vi "Host Application (Main).vi"() -> ()   [LabVIEW 2015]
doc: "Shared Variable Benchmarking Utility - Allows for the programmatic benchmarking of shared variable perfomance from single host to single target."
uses:
  Type Defs/Sequence Parameters.ctl
  Type Defs/Target Type.ctl
  Type Defs/Variable Data Type.ctl
  Type Defs/Target Config Cluster.ctl
  Type Defs/RT Target Type.ctl
  Type Defs/Control Refs.ctl
  SV B-M (Host) Class/SV B-M (Host).lvclass
panel:
  in  "Tab Control":T1(tab)=enum."Benchmark Utility"
  in  "Abort Config":bool
  in  "Run Config":bool
  out "Config Console":string="Waiting..."
  in  "Targets to Configure":T2[](array[typedef])
  out "Test #":string
  in  "Load":bool
  in  "Save":bool
  in  "Delete":bool
  in  "Copy":bool
  in  "Insert After":bool
  in  "Insert Before":bool
  in  "Seq Parameters":T4[](array[typedef]) {"# of Variables per Library" items=["50"=50, "100"=100, "150"=150, "200"=200, "250"=250, "300"=300, "350"=350, "400"=400, "450"=450, "500"=500]; "Delta" min=50 max=1000000 step=50; "Ceiling" min=50 max=1000000 step=50; "Floor" min=50 max=1000000 step=50}
  in  "Abort BM":bool
  in  "Run BM":bool
  out "Test in Progress :":string
  in  "MC Listbox":i32(listbox)=-1
  in  "Load":bool
  in  "Sequence Directory":path
  out "Config Params":T4[](array[typedef]) {"# of Variables per Library" items=["50"=50, "100"=100, "150"=150, "200"=200, "250"=250, "300"=300, "350"=350, "400"=400, "450"=450, "500"=500]; "Delta" min=50 max=1000000 step=50; "Ceiling" min=50 max=1000000 step=50; "Floor" min=50 max=1000000 step=50}
  out "CPU Load Data":cluster{dbl[], dbl[]}(graph)
  # "Shared Variable Benchmarking Utility"
  # "Target IP Address"
  # "Target Type"
  # "Username"
  # "Password"
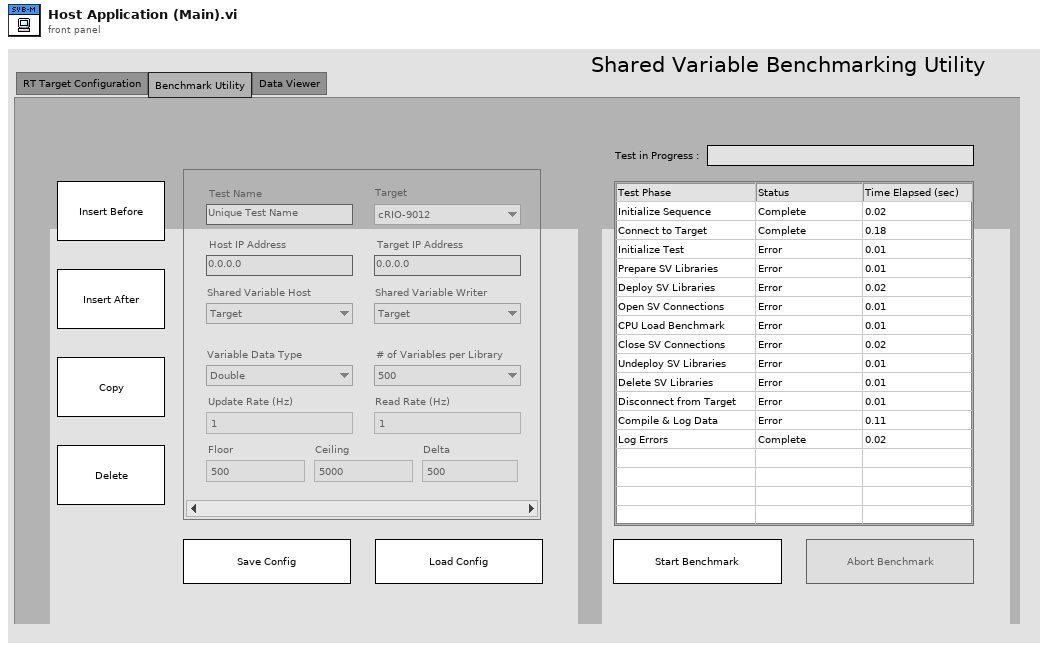
[diagram p1: front panel]
types:
  T1 = enum32{"RT Target Configuration", "Benchmark Utility", "Data Viewer"}
  T2 = typedef "Target Config Cluster.ctl" = cluster{"IP Address":string, "Target":T3, "Username":string, "Password":string}
  T3 = typedef "RT Target Type.ctl" = enum16{"cRIO-9012", "cRIO-9014", "cRIO-9022", "cRIO-9023", "cRIO-9024", "cRIO-9025", "cRIO-9068", "cRIO-9073", "cRIO-9074", "cRIO-9075", "cRIO-9076", "cRIO-9081", "cRIO-9082", "myRIO-1900", "myRIO-1950", "PXI-8101", "PXI-8115", "PXI-8119", "PXI-8820", "PXIe-8100", "PXIe-8101", "PXIe-8133", "PXIe-8135", "PXIe-8820", "sbRIO-9605", "sbRIO-9606", "sbRIO-9623", "sbRIO-9626", "sbRIO-9633", "sbRIO-9636", "Unlisted (Linux-RT)", "Unlisted (PharLap)", "Unlisted (VxWorks)"}
  T4 = typedef "Sequence Parameters.ctl" = cluster{"Test Name":string, "Target":T5, "Host IP Address":string, "Target IP Address":string, "Shared Variable Host":enum16{"Target", "Host"}, "Shared Variable Writer":enum16{"Target", "Host"}, "Variable Data Type":T6, "# of Variables per Library":u16, "Update Rate (Hz)":dbl, "Read Rate (Hz)":dbl, "Floor":u32, "Ceiling":u32, "Delta":u32}
  T5 = typedef "Target Type.ctl" = enum16{"cRIO-9012", "cRIO-9014", "cRIO-9022", "cRIO-9023", "cRIO-9024", "cRIO-9025", "cRIO-9068", "cRIO-9073", "cRIO-9074", "cRIO-9075", "cRIO-9076", "cRIO-9081", "cRIO-9082", "myRIO-1900", "myRIO-1950", "PXI-8101", "PXI-8115", "PXI-8119", "PXI-8820", "PXIe-8100", "PXIe-8101", "PXIe-8133", "PXIe-8135", "PXIe-8820", "sbRIO-9605", "sbRIO-9606", "sbRIO-9623", "sbRIO-9626", "sbRIO-9633", "sbRIO-9636", "Unlisted (Linux-RT)", "Unlisted (PharLap)", "Unlisted (VxWorks)", "Windows Target"}
  T6 = typedef "Variable Data Type.ctl" = enum16{"U8", "U16", "U32", "U64", "I8", "I16", "I32", "I64", "Single", "Double", "Boolean", "String"}
  T7 = enum16{"BM Init", "BM Run", "BM End", "Config Init", "Config Run", "Config End"}
  T8 = typedef "Control Refs.ctl" = cluster{"Save":refnum<vi>, "Load":refnum<vi>, "Delete":refnum<vi>, "Copy":refnum<vi>, "Insert Before":refnum<vi>, "Insert After":refnum<vi>, "Run BM":refnum<vi>, "Abort BM":refnum<vi>, "Run Config":refnum<vi>, "Abort Config":refnum<vi>, "Seq Parameters":refnum<vi>, "Target Config":refnum<vi>}
  T9 = typedef "Sequence Parameters Ref.ctl" = refnum<vi>
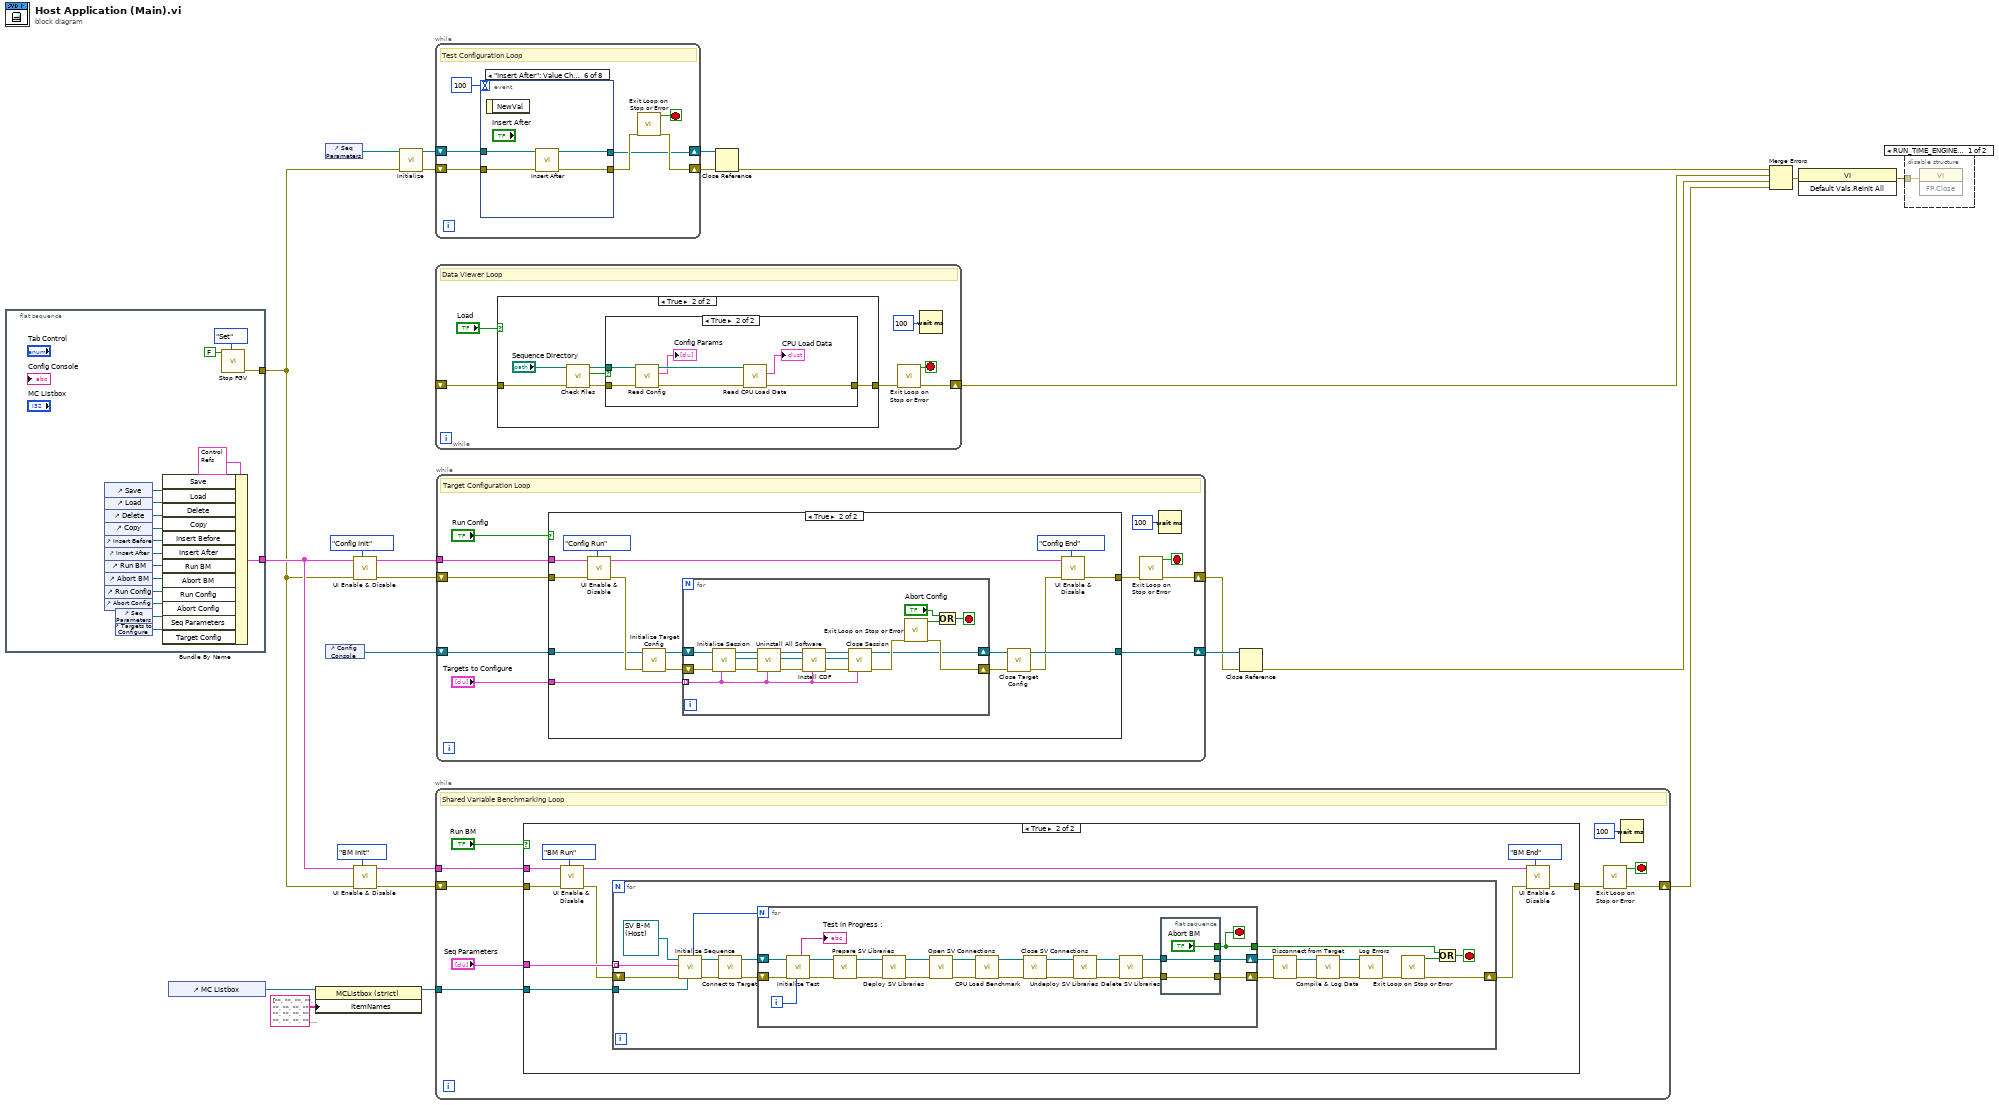
[diagram p0: block diagram]
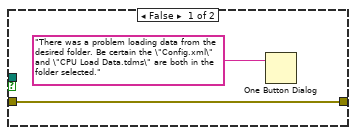
[diagram p3: hidden frame]
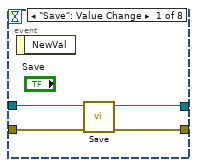
[diagram p7: hidden frame]
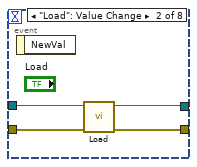
[diagram p8: hidden frame]
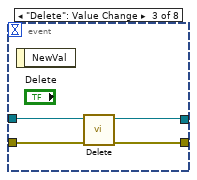
[diagram p9: hidden frame]
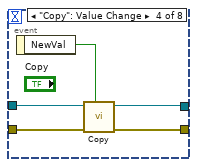
[diagram p10: hidden frame]
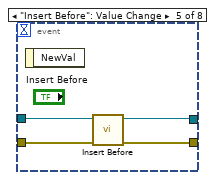
[diagram p11: hidden frame]
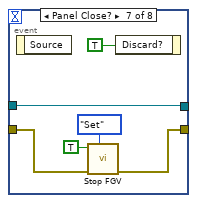
[diagram p12: hidden frame]
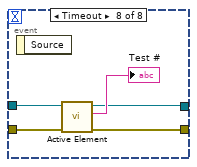
[diagram p13: hidden frame]
diagram:
  n1 = flat-sequence {
    tunnel: [w27] -> w4
    tunnel: [w26] -> w14
    frame #0 {
      n2 = control-ref of="Save"() -> (w40:refnum<vi>)
      n3 = control-ref of="Load"() -> (w39:refnum<vi>)
      n4 = control-ref of="Delete"() -> (w38:refnum<vi>)
      n5 = control-ref of="Copy"() -> (w37:refnum<vi>)
      n6 = control-ref of="Insert Before"() -> (w36:refnum<vi>)
      n7 = control-ref of="Insert After"() -> (w35:refnum<vi>)
      n8 = control-ref of="Run BM"() -> (w34:refnum<vi>)
      n9 = control-ref of="Abort BM"() -> (w33:refnum<vi>)
      n10 = control-ref of="Run Config"() -> (w32:refnum<vi>)
      n11 = control-ref of="Abort Config"() -> (w31:refnum<vi>)
      n12 = control-ref of="Seq Parameters"() -> (w30:refnum<vi>)
      n13 = control-ref of="Targets to Configure"() -> (w28:refnum<vi>)
      n14 = Bundle By Name(cluster=T8 {"Save"=refnum, "Load"=refnum, "Delete"=refnum, "Copy"=refnum, "Insert Before"=refnum, "Insert After"=refnum, "Run BM"=refnum, "Abort BM"=refnum, "Run Config"=refnum, "Abort Config"=refnum, "Seq Parameters"=refnum, "Target Config"=refnum} ("Cluster"), "Save"=w40, "Load"=w39, "Delete"=w38, "Copy"=w37, "Insert Before"=w36, "Insert After"=w35, "Run BM"=w34, "Abort BM"=w33, "Run Config"=w32, "Abort Config"=w31, "Seq Parameters"=w30, "Target Config"=w28) -> (w26:T8)
      n15 = call "Stop FGV.vi"("Mode"=enum16{"Set", "Get"}."Set", "Set Stop Condition"=FALSE) -> ("error out (no error)"=w27:errorcluster)  [unwired: 8 in, 1 out]
    }
  }
  n16 = control-ref of="MC Listbox"() -> (w8:refnum<vi>)
  n17 = property class="MCListbox (strict)"(reference=w8, "ItemNames"=string[][] [["", "", "", "", "", "", "", "", "", "", "", "", "", "", "", "", "", "", "", "", ""], ["", "", "", "", "", "", "", "", "", "", "", "", "", "", "", "", "", "", "", "", ""], ["", "", "", "", "", "", "", "", "", "", "", "", "", "", "", "", "", "", "", "", ""], ["", "", "", "", "", "", "", "", "", "", "", "", "", "", "", "", "", "", "", "", ""], ["", "", "", "", "", "", "", "", "", "", "", "", "", "", "", "", "", "", "", "", ""], ["", "", "", "", "", "", "", "", "", "", "", "", "", "", "", "", "", "", "", "", ""], ["", "", "", "", "", "", "", "", "", "", "", "", "", "", "", "", "", "", "", "", ""], ["", "", "", "", "", "", "", "", "", "", "", "", "", "", "", "", "", "", "", "", ""], ["", "", "", "", "", "", "", "", "", "", "", "", "", "", "", "", "", "", "", "", ""], ["", "", "", "", "", "", "", "", "", "", "", "", "", "", "", "", "", "", "", "", ""], ["", "", "", "", "", "", "", "", "", "", "", "", "", "", "", "", "", "", "", "", ""], ["", "", "", "", "", "", "", "", "", "", "", "", "", "", "", "", "", "", "", "", ""], ["", "", "", "", "", "", "", "", "", "", "", "", "", "", "", "", "", "", "", "", ""], ["", "", "", "", "", "", "", "", "", "", "", "", "", "", "", "", "", "", "", "", ""], ["", "", "", "", "", "", "", "", "", "", "", "", "", "", "", "", "", "", "", "", ""], ["", "", "", "", "", "", "", "", "", "", "", "", "", "", "", "", "", "", "", "", ""], ["", "", "", "", "", "", "", "", "", "", "", "", "", "", "", "", "", "", "", "", ""], ["", "", "", "", "", "", "", "", "", "", "", "", "", "", "", "", "", "", "", "", ""], ["", "", "", "", "", "", "", "", "", "", "", "", "", "", "", "", "", "", "", "", ""], ["", "", "", "", "", "", "", "", "", "", "", "", "", "", "", "", "", "", "", "", ""], ["", "", "", "", "", "", "", "", "", "", "", "", "", "", "", "", "", "", "", "", "."]] ("Item Names")) -> (reference out=w6:refnum<vi>)  [unwired: 1 in, 1 out]
  n18 = control-ref of="Config Console"() -> (w13:refnum<vi>)
  n19 = control-ref of="Seq Parameters"() -> (w5:refnum<vi>)
  n20 = call "UI Enable & Disable.vi"("Mode"=T7."Config Init", "error in (no error)"=w4, "Ctl Refs In"=w14) -> ("error out"=w15:errorcluster, "Ctl Refs Out"=w16:T8)  [unwired: 7 in]
  n21 = call "UI Enable & Disable.vi"("Mode"=T7."BM Init", "error in (no error)"=w4, "Ctl Refs In"=w14) -> ("error out"=w20:errorcluster, "Ctl Refs Out"=w18:T8)  [unwired: 7 in]
  n22 = call "Initialize.vi"("error in (no error)"=w4, "Test Configs In"=w5) -> ("error out"=w25:errorcluster, "Test Configs Out"=w22:T9)  [unwired: 8 in]
  n23 = while {
    shift-right: [w46] -> w24
    shift-left: w25 -> [w49]
    shift-right: [w43] -> w21
    shift-left: w22 -> [w44]
    stop <- w45 stop-if-true
    # "Test Configuration Loop"
    n24 = event shown="[5] \"Insert After\": Value Change" {
      selector: _ -> [_ _ _ _ _ _ _ _]
      dyn-events: _ -> [_ _ _ _ _ _ _ _]
      timeout: 100 -> [_ _ _ _ _ _ _ _]
      tunnel: w49 -> [w53 w57 w61 w66 w70 w74 w79 w85]
      tunnel: [w52 w56 w60 w65 w69 w73 w78 w84] -> w47
      tunnel: w44 -> [w51 w55 w59 w63 w68 w72 w75 w82]
      tunnel: [w50 w54 w58 w62 w67 w71 w75 w81] -> w43
      event "Save": Value Change {
        n25 = event-data() -> ()  [unwired: 1 in, 1 out]
        n26 = call "Save.vi"("error in (no error)"=w53, "Test Configs In"=w51) -> ("error out"=w52:errorcluster, "Test Configs Out"=w50:T9)  [unwired: 8 in]
      }
      event "Load": Value Change {
        n27 = event-data() -> ()  [unwired: 1 in, 1 out]
        n28 = call "Load.vi"("error in (no error)"=w57, "Test Configs In"=w55) -> ("error out"=w56:errorcluster, "Test Configs Out"=w54:T9)  [unwired: 8 in]
      }
      event "Delete": Value Change {
        n29 = event-data() -> ()  [unwired: 1 in, 1 out]
        n30 = call "Delete.vi"("error in (no error)"=w61, "Test Configs In"=w59) -> ("error out"=w60:errorcluster, "Test Configs Out"=w58:T9)  [unwired: 8 in]
      }
      event "Copy": Value Change {
        n31 = event-data() -> ("NewVal"=w64:bool)  [unwired: 1 in]
        n32 = call "Copy.vi"("Copy Enabled?"=w64, "error in (no error)"=w66, "Test Configs In"=w63) -> ("error out"=w65:errorcluster, "Test Configs Out"=w62:T9)  [unwired: 7 in]
      }
      event "Insert Before": Value Change {
        n33 = event-data() -> ()  [unwired: 1 in, 1 out]
        n34 = call "Insert Before.vi"("error in (no error)"=w70, "Test Configs In"=w68) -> ("error out"=w69:errorcluster, "Test Configs Out"=w67:T9)  [unwired: 8 in]
      }
      event "Insert After": Value Change {
        n35 = event-data() -> ()  [unwired: 1 in, 1 out]
        n36 = call "Insert After.vi"("error in (no error)"=w74, "Test Configs In"=w72) -> ("error out"=w73:errorcluster, "Test Configs Out"=w71:T9)  [unwired: 8 in]
      }
      event Panel Close? {
        n37 = event-data() -> ()  [unwired: 1 in, 1 out]
        n38 = call "Stop FGV.vi"("Mode"=enum16{"Set", "Get"}."Set", "error in (no error)"=w79, "Set Stop Condition"=TRUE) -> ("error out (no error)"=w78:errorcluster)  [unwired: 7 in, 1 out]
        n39 = event-data("Discard?"=TRUE) -> ()  [unwired: 1 in, 1 out]
      }
      event Timeout {
        n40 = event-data() -> ()  [unwired: 1 in, 1 out]
        n41 = call "Active Element.vi"("error in (no error)"=w85, "Test Configs In"=w82) -> ("error out"=w84:errorcluster, "Active Test"=→"Test #":string, "Test Configs Out"=w81:T9)  [unwired: 7 in]
      }
    }
    n42 = call "Exit Loop on Stop or Error.vi"("error in (no error)"=w47) -> ("error out"=w46:errorcluster, "Exit?"=w45:bool)  [unwired: 9 in]
  }
  n43 = while {
    shift-right: [w87] -> w1
    shift-left: _ -> [w90]
    stop <- w88 stop-if-true
    # "Data Viewer Loop"
    n44 = case shown="True" "Load" {
      tunnel: w90 -> [w92 w97]
      tunnel: [w92 w98] -> w89
      frame False {
      }
      frame True {
        n45 = call "Check Files.vi"("error in (no error)"=w97, "Sequence Directory In"="Sequence Directory") -> ("error out"=w95:errorcluster, "Files Valid?"=w94:bool, "Sequence Directory Out"=w93:path)  [unwired: 7 in]
        n46 = case shown="True" w94 {
          tunnel: [w100 w106] -> w98
          tunnel: w95 -> [w100 w105]
          tunnel: w93 -> [_ w104]
          frame False {
            n47 = One Button Dialog(message="There was a problem loading data from the desired folder. Be certain the \"Config.xml\" and \"CPU Load Data.tdms\" are both in the folder selected.") -> ()  [unwired: 1 in, 1 out]
          }
          frame True {
            n48 = call "Read Config.vi"("error in (no error)"=w105, "Sequence Directory"=w104) -> ("error out"=w107:errorcluster, "Sequence Parameters"=→"Config Params":T4[], "Sequence Directory Out"=w103:path)  [unwired: 7 in]
            n49 = call "Read CPU Load Data.vi"("error in (no error)"=w107, "Sequence Directory In"=w103) -> ("error out"=w106:errorcluster, "XY Graph Data"=→"CPU Load Data":cluster{dbl[], dbl[]})  [unwired: 7 in, 1 out]
          }
        }
      }
    }
    n50 = call "Exit Loop on Stop or Error.vi"("error in (no error)"=w89) -> ("error out"=w87:errorcluster, "Exit?"=w88:bool)  [unwired: 9 in]
    n51 = Wait (ms)(milliseconds to wait=u32 100) -> ()  [unwired: 1 out]
  }
  n52 = while {
    shift-right: [w108] -> w10
    shift-left: w20 -> [w115]
    tunnel: w18 -> [w112]
    tunnel: w6 -> [w110]
    stop <- w113 stop-if-true
    # "Shared Variable Benchmarking Loop"
    n53 = case shown="True" "Run BM" {
      tunnel: w115 -> [w117 w127]
      tunnel: w112 -> [_ w126]
      tunnel: "Seq Parameters" -> [_ w122]
      tunnel: w110 -> [_ w120]
      tunnel: [w117 w118] -> w109
      frame False {
      }
      frame True {
        n54 = call "UI Enable & Disable.vi"("Mode"=T7."BM Run", "error in (no error)"=w127, "Ctl Refs In"=w126) -> ("error out"=w121:errorcluster, "Ctl Refs Out"=w124:T8)  [unwired: 7 in]
        n55 = for {
          tunnel: w122 -> [w147] mode=indexing
          shift-right: [w143] -> w119
          shift-left: w121 -> [w146]
          tunnel: w120 -> [w144]
          stop <- w141 stop-if-true
          n56 = call "Initialize Sequence.vi"("Listbox Ref In"=w144, "error in (no error)"=w146, "Seq Parameters"=w147, "SV B-M in"=refnum<class "SV B-M (Host).lvclass"> refnum ("SV B-M.lvclass")) -> ("error out"=w137:errorcluster, "SV B-M out"=w139:refnum<class "SV B-M (Host).lvclass">, "# of Tests"=w140:i32)  [unwired: 5 in]
          n57 = call "Connect to Target.vi"("error in (no error)"=w137, "SV B-M (Host) in"=w139) -> ("error out"=w136:errorcluster, "SV B-M (Host) out"=w138:refnum<class "SV B-M (Host).lvclass">)  [unwired: 8 in]
          n58 = for {
            N: w140 -> [_]
            shift-right: [w149] -> w133
            shift-left: w136 -> [w170]
            shift-right: [w151] -> w134
            shift-left: w138 -> [w169]
            tunnel: [w148] -> w132
            i -> [w167]
            stop <- w148 stop-if-true
            n59 = call "Initialize Test.vi"("Test Index"=w167, "error in (no error)"=w170, "SV B-M in"=w169) -> ("error out"=w165:errorcluster, "SV B-M out"=w166:refnum<class "SV B-M (Host).lvclass">, "Test In Progress"=→"Test in Progress :":string)  [unwired: 6 in]
            n60 = call "Prepare SV Libraries.vi"("error in (no error)"=w165, "SV B-M in"=w166) -> ("error out"=w163:errorcluster, "SV B-M out"=w164:refnum<class "SV B-M (Host).lvclass">)  [unwired: 8 in]
            n61 = call "Deploy SV Libraries.vi"("error in (no error)"=w163, "SV B-M in"=w164) -> ("error out"=w159:errorcluster, "SV B-M out"=w160:refnum<class "SV B-M (Host).lvclass">)  [unwired: 8 in]
            n62 = call "Open SV Connections.vi"("error in (no error)"=w159, "SV B-M (Host) in"=w160) -> ("error out"=w155:errorcluster, "SV B-M (Host) out"=w156:refnum<class "SV B-M (Host).lvclass">)  [unwired: 8 in]
            n63 = call "CPU Load Benchmark.vi"("error in (no error)"=w155, "SV B-M (Host) in"=w156) -> ("error out"=w153:errorcluster, "SV B-M (Host) out"=w154:refnum<class "SV B-M (Host).lvclass">)  [unwired: 8 in]
            n64 = call "Close SV Connections.vi"("error in (no error)"=w153, "SV B-M (Host) in"=w154) -> ("error out"=w157:errorcluster, "SV B-M (Host) out"=w158:refnum<class "SV B-M (Host).lvclass">)  [unwired: 8 in]
            n65 = call "Undeploy SV Libraries.vi"("error in (no error)"=w157, "SV B-M in"=w158) -> ("error out"=w161:errorcluster, "SV B-M out"=w162:refnum<class "SV B-M (Host).lvclass">)  [unwired: 8 in]
            n66 = call "Delete SV Libraries.vi"("error in (no error)"=w161, "SV B-M (Host) in"=w162) -> ("error out"=w150:errorcluster, "SV B-M (Host) out"=w152:refnum<class "SV B-M (Host).lvclass">)  [unwired: 8 in]
            n67 = flat-sequence {
              tunnel: ["Abort BM"] -> w148
              tunnel: w152 -> [w172]
              tunnel: [w172] -> w151
              tunnel: [w171] -> w149
              tunnel: w150 -> [w171]
              frame #0 {
              }
            }
          }
          n68 = call "Disconnect from Target.vi"("error in (no error)"=w133, "SV B-M (Host) in"=w134) -> ("error out"=w131:errorcluster, "SV B-M (Host) out"=w130:refnum<class "SV B-M (Host).lvclass">)  [unwired: 8 in]
          n69 = call "Compile & Log Data.vi"("error in (no error)"=w131, "SV B-M (Host) in"=w130) -> ("error out"=w128:errorcluster, "SV B-M (Host) out"=w129:refnum<class "SV B-M (Host).lvclass">)  [unwired: 8 in]
          n70 = call "Log Errors.vi"("error in (no error)"=w128, "SV B-M (Host) in"=w129) -> ("error out"=w135:errorcluster)  [unwired: 9 in]
          n71 = call "Exit Loop on Stop or Error.vi"("error in (no error)"=w135) -> ("error out"=w143:errorcluster, "Exit?"=w142:bool)  [unwired: 9 in]
          n72 = Or(x=w132, y=w142) -> (x .or. y?=w141:bool)
        }
        n73 = call "UI Enable & Disable.vi"("Mode"=T7."BM End", "error in (no error)"=w119, "Ctl Refs In"=w124) -> ("error out"=w118:errorcluster)  [unwired: 7 in, 1 out]
      }
    }
    n74 = call "Exit Loop on Stop or Error.vi"("error in (no error)"=w109) -> ("error out"=w108:errorcluster, "Exit?"=w113:bool)  [unwired: 9 in]
    n75 = Wait (ms)(milliseconds to wait=u32 100) -> ()  [unwired: 1 out]
  }
  n76 = while {
    shift-right: [w178] -> w11
    shift-left: w15 -> [w183]
    tunnel: w16 -> [w180]
    shift-right: [w174] -> w12
    shift-left: w13 -> [w176]
    stop <- w181 stop-if-true
    # "Target Configuration Loop"
    n77 = case shown="True" "Run Config" {
      tunnel: w183 -> [w185 w200]
      tunnel: w180 -> [_ w199]
      tunnel: [w185 w195] -> w179
      tunnel: w176 -> [w184 w192]
      tunnel: "Targets to Configure" -> [_ w190]
      tunnel: [w184 w187] -> w174
      frame False {
      }
      frame True {
        n78 = call "UI Enable & Disable.vi"("Mode"=T7."Config Run", "error in (no error)"=w200, "Ctl Refs In"=w199) -> ("error out"=w194:errorcluster, "Ctl Refs Out"=w197:T8)  [unwired: 7 in]
        n79 = call "Initialize Target Config.vi"("error in (no error)"=w194, "Console Ref In"=w192) -> ("error out"=w193:errorcluster, "Console Ref Out"=w191:refnum<vi>)  [unwired: 8 in]
        n80 = for {
          shift-right: [w218] -> w188
          shift-left: w193 -> [w207]
          shift-right: [w201] -> w189
          shift-left: w191 -> [w208]
          tunnel: w190 -> [w203] mode=indexing
          stop <- w216 stop-if-true
          n81 = call "Initialize Session.vi"("Target Config"=w203, "error in (no error)"=w207, "Console Ref In"=w208) -> ("error out"=w206:errorcluster, "Sys Cfg Session Out"=w213:refnum<k21>, "Console Ref Out"=w214:refnum<vi>)  [unwired: 6 in]
          n82 = call "Uninstall All Software.vi"("Target Config"=w203, "error in (no error)"=w206, "Sys Cfg Session In"=w213, "Console Ref In"=w214) -> ("error out"=w205:errorcluster, "Sys Cfg Session Out"=w209:refnum<k21>, "Console Ref Out"=w210:refnum<vi>)  [unwired: 5 in]
          n83 = call "Install CDF.vi"("Target Config"=w203, "error in (no error)"=w205, "Sys Cfg Session In"=w209, "Console Ref In"=w210) -> ("error out"=w204:errorcluster, "Sys Cfg Session Out"=w211:refnum<k21>, "Console Ref Out"=w212:refnum<vi>)  [unwired: 5 in]
          n84 = call "Close Session.vi"("Target Config"=w203, "error in (no error)"=w204, "Sys Cfg Session In"=w211, "Console Ref In"=w212) -> ("error out"=w202:errorcluster, "Console Ref Out"=w201:refnum<vi>)  [unwired: 6 in]
          n85 = call "Exit Loop on Stop or Error.vi"("error in (no error)"=w202) -> ("error out"=w218:errorcluster, "Exit?"=w217:bool)  [unwired: 9 in]
          n86 = Or(x="Abort Config", y=w217) -> (x .or. y?=w216:bool)
        }
        n87 = call "Close Target Config.vi"("error in (no error)"=w188, "Console Ref In"=w189) -> ("error out"=w186:errorcluster, "Console Ref Out"=w187:refnum<vi>)  [unwired: 8 in]
        n88 = call "UI Enable & Disable.vi"("Mode"=T7."Config End", "error in (no error)"=w186, "Ctl Refs In"=w197) -> ("error out"=w195:errorcluster)  [unwired: 7 in, 1 out]
      }
    }
    n89 = call "Exit Loop on Stop or Error.vi"("error in (no error)"=w179) -> ("error out"=w178:errorcluster, "Exit?"=w181:bool)  [unwired: 9 in]
    n90 = Wait (ms)(milliseconds to wait=u32 100) -> ()  [unwired: 1 out]
  }
  n91 = Close Reference(reference=w21, error in (no error)=w24) -> (error out=w3:errorcluster)
  n92 = Close Reference(reference=w12, error in (no error)=w11) -> (error out=w2:errorcluster)
  n93 = Merge Errors(w3, w1, w2, w10) -> (w9:errorcluster)
  n94 = invoke class="VI" method="Default Vals.Reinit All"(error in=w9) -> (error out=w23:errorcluster)  [unwired: 2 in, 2 out]
  n95 = disable-structure shown="RUN_TIME_ENGINE==True" {
    disable-tunnel: w23 -> [w219 _]
    frame condition #0 {
      n96 = invoke class="VI" method="FP.Close"(error in=w219) -> ()  [unwired: 2 in, 3 out]
    }
    frame condition #1 (active) {
    }
  }
